vi "Updater Convert TDMS Test Runs 4.3 to 5.0 Prompted Inputs.vi"(7 "Source TDMS File In":refnum<k34>, 8 "error in (no error)":errorcluster, 10 "Group Name In":string, 11 "New TDMS File In":refnum<k34>) -> (0 "error out":errorcluster, 2 "Group Name Out":string, 3 "New TDMS File Out":refnum<k34>, 5 "Source TDMS File Out":refnum<k34>)   [LabVIEW 2011]
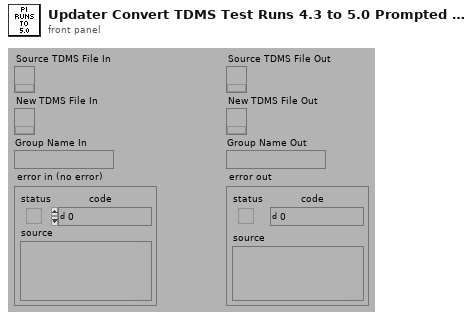
[diagram p1: front panel]
types:
  T1 = typedef "PI Channel Type.ctl" = enum16{"Data", "Limit", "Invalid"}
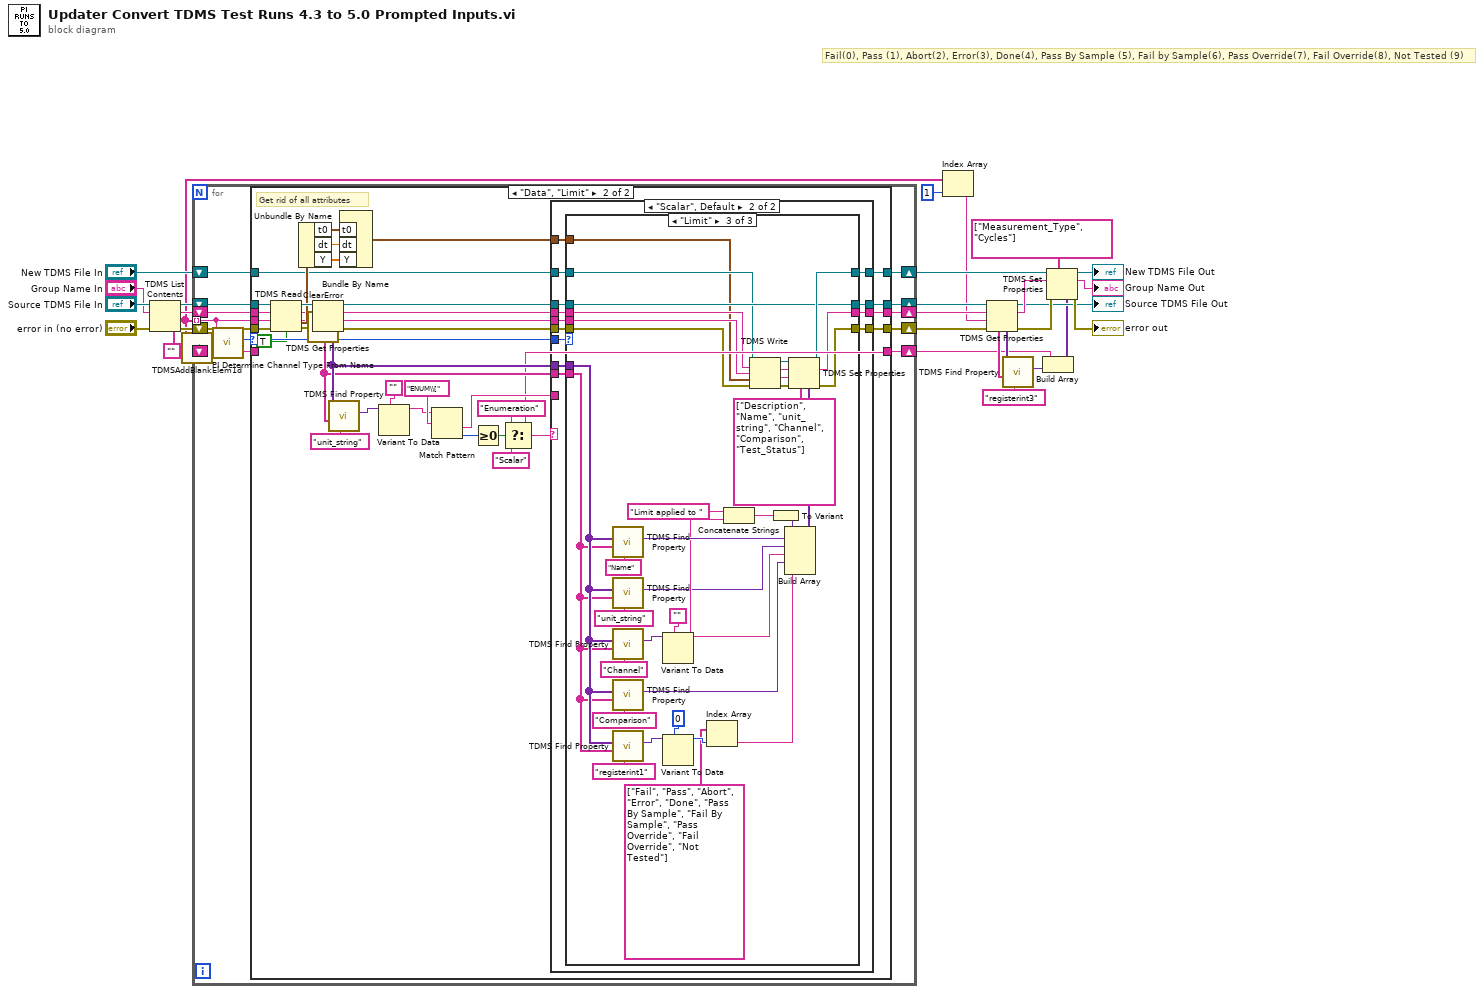
[diagram p0: block diagram]
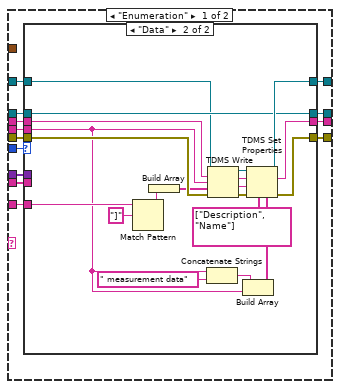
[diagram p3: hidden frame]
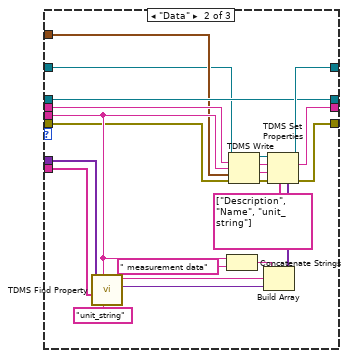
[diagram p6: hidden frame]
diagram:
  # "Fail(0), Pass (1), Abort(2), Error(3), Done(4), Pass By Sample (5), Fail by Sample(6), Pass Override(7), Fail Override(8), Not Tested (9)"
  n1 = TDMS List Contents(4:"error in (no error)", 6:"Group Name In", 7:"Source TDMS File In") -> (0:w26:errorcluster, 1:w1:string[], 2:w24:string, 3:w25:refnum<k34>)
  n2 = call <vilib>:"TDMSAddBlankElem1d.vi"("input string array"=w1) -> ("output string array with blank element at the beginning"=w4:string[])
  n3 = for {
    shift-right: [w40] -> w13
    shift-left: w26 -> [w37]
    shift-right: [w41] -> w23
    shift-left: w25 -> [w36]
    tunnel: w4 -> [w34] mode=indexing
    shift-right: [w39] -> w22
    shift-left: w24 -> [w35]
    shift-right: [w38] -> w14
    shift-left: "New TDMS File In" -> [w33]
    shift-right: [w31] -> w5
    shift-left: "" -> [w30]
    n4 = call "PI Determine Channel Type From Name.vi"("Channel Name"=w34) -> ("Channel Type"=w32:T1)  [unwired: 10 out]
    n5 = case shown="\"Data\", \"Limit\"" w32 {
      selector: w32 -> [_ w68]
      tunnel: [w46 w84] -> w41
      tunnel: [w43 w83] -> w40
      tunnel: [w45 w82] -> w39
      tunnel: [w44 w81] -> w38
      tunnel: w37 -> [w43 w76]
      tunnel: w36 -> [w46 w74]
      tunnel: w35 -> [w45 w73]
      tunnel: w34 -> [_ w72]
      tunnel: w33 -> [w44 w49]
      tunnel: [w42 w54] -> w31
      tunnel: w30 -> [w42 _]
      frame "Invalid" {
        # "Empty channel for Group level"
      }
      frame "Data", "Limit" {
        # "Get rid of all attributes"
        n6 = TDMS Read(0:w74, 5:w73, 7:w72, 11:w76, 13:TRUE ("return channels in file order? (F)")) -> (4:w75:refnum<k34>, 6:w52:string, 8:w51:string, 10:w71:waveform(dbl), 15:w48:errorcluster)  [unwired: 3 in, 1 out]
        n7 = Unbundle By Name(w71) -> ("t0"=w70:timestamp, "dt"=w69:dbl, "Y"=w67:dbl[])
        n8 = call <vilib>:"ClearError.vi"("error in (no error)"=w48) -> ("error out"=w50:errorcluster)
        n9 = TDMS Get Properties(8:w50, 9:w51, 10:w52, 11:w75) -> (0:w80:errorcluster, 1:w79:string, 2:w78:string, 3:w77:refnum<k34>, 4:w57:variant[], 6:w56:string[])  [unwired: 2 out]
        n10 = call "TDMS Find Property.vi"("Property Name"="unit_string", "Property Names"=w56, "Property Values"=w57) -> ("Property Value"=w59:variant)  [unwired: 5 out]
        n11 = Bundle By Name("t0"=w70, "dt"=w69, "Y"=w67) -> (w53:waveform(dbl))  [unwired: 1 out]
        n12 = Variant To Data(type="", Variant=w59) -> (data=w61:string)  [unwired: 1 in, 1 out]
        n13 = Match Pattern(string=w61, regular expression="ENUM\\[") -> (after substring=w55:string, offset past match=w64:i32)  [unwired: 3 out]
        n14 = Greater Or Equal To 0?(x=w64) -> (x >= 0?=w63:bool)
        n15 = Select(t="Enumeration", s=w63, f="Scalar") -> (s? t:f=w54:string)
        n16 = case shown="\"Scalar\", Default" w54 {
          tunnel: [w97 w134] -> w84
          tunnel: [w96 w133] -> w83
          tunnel: [w95 w132] -> w82
          tunnel: [w94 w131] -> w81
          tunnel: w80 -> [w93 w130]
          tunnel: w79 -> [w92 w129]
          tunnel: w78 -> [w91 w128]
          tunnel: w77 -> [w90 w127]
          tunnel: w49 -> [w89 w126]
          tunnel: w68 -> [w88 w125]
          tunnel: w57 -> [w87 w124]
          tunnel: w56 -> [w86 w123]
          tunnel: w55 -> [w85 _]
          tunnel: w53 -> [_ w122]
          frame "Enumeration" {
            n17 = case shown="\"Data\"" w88 {
              tunnel: w93 -> [w100 w111]
              tunnel: w91 -> [w99 w109]
              tunnel: w90 -> [w101 w118]
              tunnel: [w101 w118] -> w97
              tunnel: [w100 w119] -> w96
              tunnel: w92 -> [_ w108]
              tunnel: [w99 w120] -> w95
              tunnel: w89 -> [w98 w105]
              tunnel: [w98 w121] -> w94
              tunnel: w86 -> [_ _]
              tunnel: w87 -> [_ _]
              tunnel: w85 -> [_ w114]
              frame "Limit", Default {
              }
              frame "Data" {
                n18 = Match Pattern(string=w114, regular expression="]") -> (before substring=w103:string)  [unwired: 4 out]
                n19 = Build Array(w103) -> (w102:string[])
                n20 = Concatenate Strings(w108, " measurement data" ("string")) -> (w112:string)
                n21 = TDMS Write(0:w105, 5:w109, 7:w108, 9:w102, 11:w111) -> (4:w104:refnum<k34>, 6:w106:string, 8:w107:string, 15:w110:errorcluster)  [unwired: 1 in]
                n22 = Build Array(w112, w108) -> (w115:string[])
                n23 = TDMS Set Properties(5:w115, 7:string[] ["Description", "Name"], 8:w110, 9:w107, 10:w106, 11:w104) -> (0:w119:errorcluster, 2:w120:string, 3:w121:refnum<k34>)  [unwired: 1 out]
              }
            }
          }
          frame "Scalar", Default {
            n24 = case shown="\"Limit\"" w125 {
              tunnel: w130 -> [w137 w145 w164]
              tunnel: w128 -> [w136 w147 w167]
              tunnel: w127 -> [w138 w156 w191]
              tunnel: [w138 w156 w191] -> w134
              tunnel: [w137 w157 w193] -> w133
              tunnel: w129 -> [_ w146 w166]
              tunnel: [w136 w158 w194] -> w132
              tunnel: w126 -> [w135 w143 w168]
              tunnel: [w135 w159 w195] -> w131
              tunnel: w123 -> [_ w149 w170]
              tunnel: w124 -> [_ w150 w171]
              tunnel: w122 -> [_ w144 w165]
              frame Default {
              }
              frame "Data" {
                n25 = call "TDMS Find Property.vi"("Property Name"="unit_string", "Property Names"=w149, "Property Values"=w150) -> ("Property Value"=w151:variant)  [unwired: 5 out]
                n26 = Concatenate Strings(w146, " measurement data" ("string")) -> (w148:string)
                n27 = TDMS Write(0:w143, 5:w147, 7:w146, 9:w144, 11:w145) -> (4:w142:refnum<k34>, 6:w141:string, 8:w140:string, 15:w139:errorcluster)  [unwired: 1 in]
                n28 = Build Array(w148, w146, w151) -> (w153:variant[])
                n29 = TDMS Set Properties(5:w153, 7:string[] ["Description", "Name", "unit_string"], 8:w139, 9:w140, 10:w141, 11:w142) -> (0:w157:errorcluster, 2:w158:string, 3:w159:refnum<k34>)  [unwired: 1 out]
              }
              frame "Limit" {
                n30 = call "TDMS Find Property.vi"("Property Name"="Name", "Property Names"=w170, "Property Values"=w171) -> ("Property Value"=w184:variant)  [unwired: 5 out]
                n31 = call "TDMS Find Property.vi"("Property Name"="unit_string", "Property Names"=w170, "Property Values"=w171) -> ("Property Value"=w169:variant)  [unwired: 5 out]
                n32 = call "TDMS Find Property.vi"("Property Name"="Channel", "Property Names"=w170, "Property Values"=w171) -> ("Property Value"=w174:variant)  [unwired: 5 out]
                n33 = call "TDMS Find Property.vi"("Property Name"="Comparison", "Property Names"=w170, "Property Values"=w171) -> ("Property Value"=w176:variant)  [unwired: 5 out]
                n34 = call "TDMS Find Property.vi"("Property Name"="registerint1", "Property Names"=w170, "Property Values"=w171) -> ("Property Value"=w180:variant)  [unwired: 5 out]
                n35 = Variant To Data(type="", Variant=w174) -> (data=w173:string)  [unwired: 1 in, 1 out]
                n36 = Variant To Data(type=0, Variant=w180) -> (data=w179:i32)  [unwired: 1 in, 1 out]
                n37 = Index Array(array=string[] ["Fail", "Pass", "Abort", "Error", "Done", "Pass By Sample", "Fail By Sample", "Pass Override", "Fail Override", "Not Tested"], index=w179) -> (element=w177:string)
                n38 = Concatenate Strings("Limit applied to " ("string"), w173) -> (w189:string)
                n39 = TDMS Write(0:w168, 5:w167, 7:w166, 9:w165, 11:w164) -> (4:w163:refnum<k34>, 6:w162:string, 8:w161:string, 15:w160:errorcluster)  [unwired: 1 in]
                n40 = To Variant(anything=w189) -> (Variant=w188:variant)
                n41 = Build Array(w188, w184, w169, w173, w176, w177) -> (w187:variant[])
                n42 = TDMS Set Properties(5:w187, 7:string[] ["Description", "Name", "unit_string", "Channel", "Comparison", "Test_Status"], 8:w160, 9:w161, 10:w162, 11:w163) -> (0:w193:errorcluster, 2:w194:string, 3:w195:refnum<k34>)  [unwired: 1 out]
              }
            }
          }
        }
      }
    }
  }
  n43 = Index Array(array=w4, index=1) -> (element=w2:string)
  n44 = TDMS Get Properties(8:w13, 9:w2, 10:w22, 11:w23) -> (0:w21:errorcluster, 2:w19:string, 3:→"Source TDMS File Out":refnum<k34>, 4:w10:variant[], 6:w11:string[])  [unwired: 1 in, 2 out]
  n45 = call "TDMS Find Property.vi"("Property Name"="registerint3", "Property Names"=w11, "Property Values"=w10) -> ("Property Value"=w8:variant)  [unwired: 5 out]
  n46 = Build Array(w5, w8) -> (w7:variant[])
  n47 = TDMS Set Properties(5:w7, 7:string[] ["Measurement_Type", "Cycles"], 8:w21, 10:w19, 11:w14) -> (0:→"error out":errorcluster, 2:→"Group Name Out":string, 3:→"New TDMS File Out":refnum<k34>)  [unwired: 2 out]
